vi "RawDataSave.vi"(8 "units":string[](array[string]), 9 "varnames":string[](array[string]), 10 "Saving Cluster":T1, 11 "Array":dbl[][](array[numeric])) -> (0 "raw data filename string":string)   [LabVIEW 2017]
doc: "Creates raw data file"
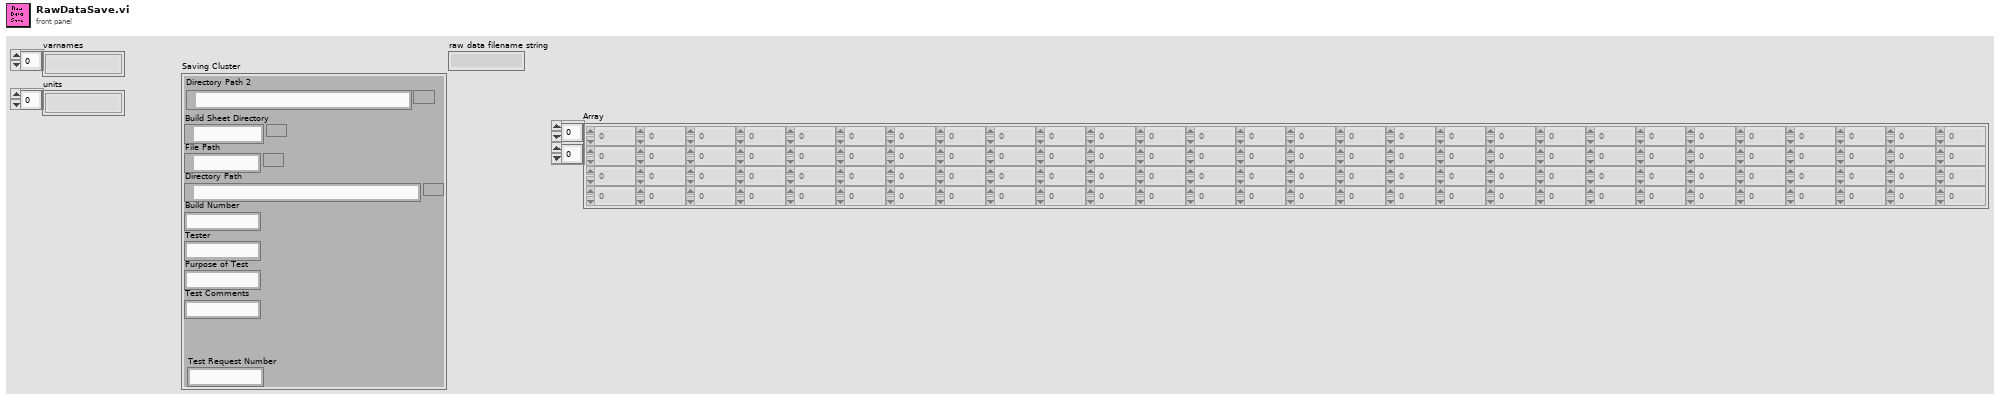
[diagram p1: front panel]
types:
  T1 = cluster{"Build Sheet Directory":path, "File Path":path, "Directory Path":path, "Build Number":string, "Tester":string, "Purpose of Test":string, "Test Comments ":string, "Test Request Number":string, "Directory Path 2":path}
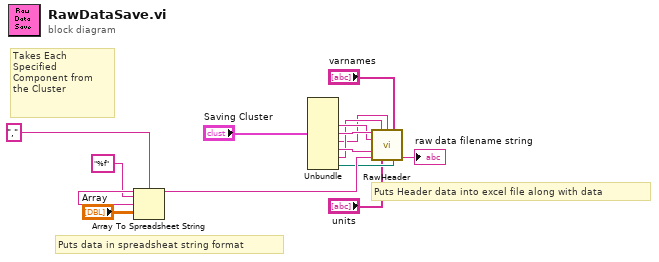
[diagram p0: block diagram]
diagram:
  # "Puts Header data into excel file along with data"
  # "Puts data in spreadsheat string format"
  # "Takes Each \nSpecified\nComponent from\nthe Cluster"
  n1 = Array To Spreadsheet String(delimiter (Tab)=",", array="Array", 3:"%f" ("delimiter (Tab)")) -> (spreadsheet string=w9:string)
  n2 = Unbundle("Saving Cluster") -> ("Build Number"=w11:string, "Tester"=w12:string, "Purpose of Test"=w2:string, "Test Comments"=w10:string, "Test Request Number"=w3:string, "Directory Path 2"=w6:path)  [unwired: 3 out]
  n3 = call "RawHeader.vi"("Tester"=w12, "test request"=w3, "purpose of test"=w2, "varnames"="varnames", "build file"=w11, "Comments on Test"=w10, "Spreadsheet Data"=w9, "units"="units", "Root Path"=w6) -> ("raw data filename string"=→"raw data filename string":string)  [unwired: 5 in, 1 out]
